vi "KM101_GetParameter.vi"(9 "Channel":i32, 10 "reference in":refnum<k7>) -> (0 "lVoltage":i32, 1 "lStepRate":i32, 2 "reference out":refnum<k7>, 3 "lStepAccn":i32)   [LabVIEW 2018, in "KIM101lib.lvlib"]
uses:
  KIM101lib.lvlib
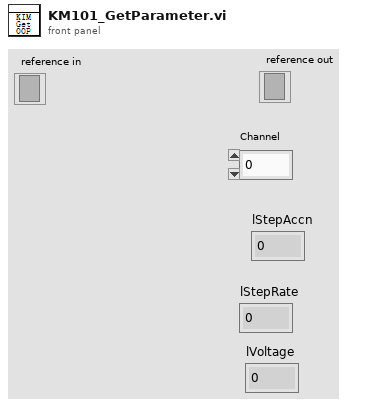
[diagram p1: front panel]
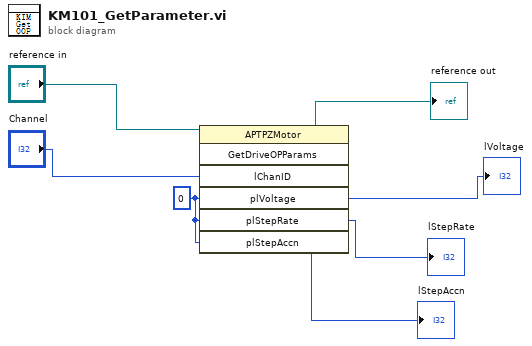
[diagram p0: block diagram]
diagram:
  w1 = 0 ("plVoltage")
  n1 = invoke class="APTPZMotor" method="GetDriveOPParams"(reference="reference in", "lChanID"="Channel", "plVoltage"=w1, "plStepRate"=w1, "plStepAccn"=w1) -> (reference out=→"reference out":refnum<k7>, "plVoltage"=→"lVoltage":i32, "plStepRate"=→"lStepRate":i32, "plStepAccn"=→"lStepAccn":i32)  [unwired: 2 in, 3 out]
